vi "Inicio_BOut.vi"(0 "Refnum in":refnum<k21>, 5 "error in (no error)":errorcluster) -> (14 "Refnum out":refnum<k21>, 19 "error out":errorcluster)   [LabVIEW 2013]
uses:
  <vilib>/DAQmx/write.llb/DAQmx Write (Digital Bool 1Line 1Point).vi
  <vilib>/DAQmx/miscellaneous.llb/DAQmx Fill In Error Info.vi
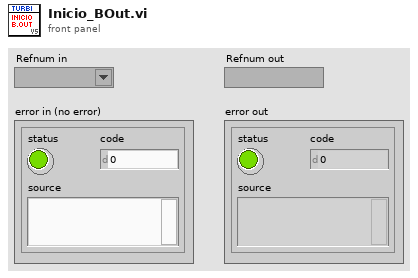
[diagram p1: front panel]
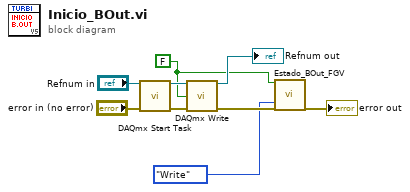
[diagram p0: block diagram]
diagram:
  w2 = FALSE ("data")
  n1 = call <vilib>:"DAQmx Start Task.vi"("task/channels in"="Refnum in", "error in"="error in (no error)") -> ("task out"=w9:refnum<k21>, "error out"=w8:errorcluster)  [unwired: 12 in]
  n2 = call-poly <vilib>:"DAQmx Write.vi"("task/channels in"=w9, "data"=w2, "error in"=w8) -> ("task out"=→"Refnum out":refnum<k21>, "error out"=w5:errorcluster)  [unwired: 10 in, 1 out]
  n3 = call "Estado_BOut_FGV.vi"("Estado IN"=w2, "Opción"=enum16{"Write", "Read"}."Write", "Error In"=w5) -> ("Error Out"=→"error out":errorcluster)  [unwired: 15 in, 1 out]
